vi "gettable2.vi"(11 "Serial Port Select":refnum<visa-resource-name>="COM3") -> (0 "COM Error":bool, 2 "Sweep Table":dbl[][](array[numeric]) format="%#_6f")   [LabVIEW 2012]
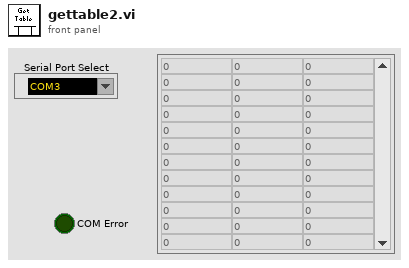
[diagram p1: front panel]
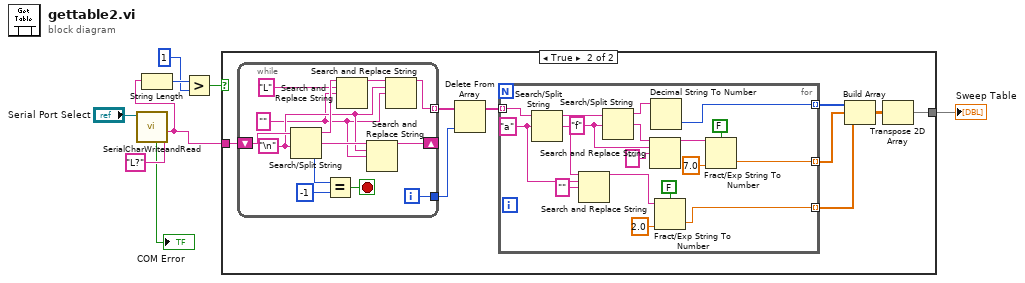
[diagram p0: block diagram]
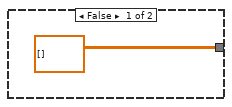
[diagram p2: hidden frame]
diagram:
  n1 = call "SerialCharWriteandRead.vi"("VISA resource name"="Serial Port Select", "write buffer"="L?") -> ("error?"=→"COM Error":bool, "read buffer"=w7:string)  [unwired: 5 in, 2 out]
  n2 = String Length(string=w7) -> (length=w5:i32)
  n3 = Greater?(x=w5, y=1) -> (0:w6:bool)
  n4 = case shown="True" w6 {
    tunnel: w7 -> [_ w18]
    tunnel: [dbl[][] [] w10] -> w1
    frame False {
    }
    frame True {
      n5 = while {
        tunnel: [w43] -> w17 mode=indexing
        shift-right: [w40] -> _
        shift-left: w18 -> [w47]
        tunnel: [w37] -> w16
        i -> [w37]
        stop <- w49 stop-if-true
        w39 = "\n"
        w38 = "" ("replace string (\"\")")
        n6 = Search/Split String(string=w47, search string/char (-)=w39) -> (substring before match=w46:string, match + rest of string=w41:string, offset of match=w42:i32)  [unwired: 1 in]
        n7 = Equal?(x=w42, y=-1) -> (x = y?=w49:bool)
        n8 = Search and Replace String(input string=w46, search string="L" ("format string"), replace string=w38) -> (result string=w44:string)  [unwired: 5 in, 3 out]
        n9 = Search and Replace String(input string=w41, search string=w39, replace string=w38) -> (result string=w40:string)  [unwired: 5 in, 3 out]
        n10 = Search and Replace String(input string=w44, search string=w39, replace string=w38) -> (result string=w43:string)  [unwired: 5 in, 3 out]
      }
      n11 = Delete From Array(array=w17, index=w16) -> (array with subset deleted=w15:string[])  [unwired: 1 in, 1 out]
      n12 = for {
        tunnel: w15 -> [w36] mode=indexing
        tunnel: [w27] -> w14 mode=indexing
        tunnel: [w23] -> w13 mode=indexing
        tunnel: [w19] -> w12 mode=indexing
        w29 = "f" ("search string/char (-)")
        w33 = "a" ("search string/char (-)")
        n13 = Search/Split String(string=w36, search string/char (-)=w33) -> (substring before match=w35:string, match + rest of string=w34:string)  [unwired: 1 in, 1 out]
        n14 = Search and Replace String(input string=w34, search string=w33, replace string="" ("replace string (\"\")")) -> (result string=w20:string)  [unwired: 5 in, 3 out]
        n15 = Search/Split String(string=w35, search string/char (-)=w29) -> (substring before match=w28:string, match + rest of string=w30:string)  [unwired: 1 in, 1 out]
        n16 = Search and Replace String(input string=w30, search string=w29, replace string="" ("replace string (\"\")")) -> (result string=w24:string)  [unwired: 5 in, 3 out]
        n17 = Decimal String To Number(string=w28) -> (number=w27:i32)  [unwired: 2 in, 1 out]
        n18 = Fract/Exp String To Number(use system decimal point (T)=FALSE, string=w20, default (0 dbl)=2.0 ("default (0 DBL)")) -> (number=w19:dbl)  [unwired: 1 in, 1 out]
        n19 = Fract/Exp String To Number(use system decimal point (T)=FALSE, string=w24, default (0 dbl)=7.0 ("default (0 DBL)")) -> (number=w23:dbl)  [unwired: 1 in, 1 out]
      }
      n20 = Build Array(w14, w13, w12) -> (w11:dbl[][])
      n21 = Transpose 2D Array(2D array=w11) -> (transposed array=w10:dbl[][])
    }
  }
  "Sweep Table" <- w1
